vi "State Enter.vi"(8 "error in":errorcluster, 11 "State Pattern in":refnum<class "State Pattern.lvclass">) -> (0 "error out":errorcluster, 3 "State Pattern out":refnum<class "State Pattern.lvclass">)   [LabVIEW 2021, in "State Pattern.lvclass"]
uses:
  State Pattern.lvclass
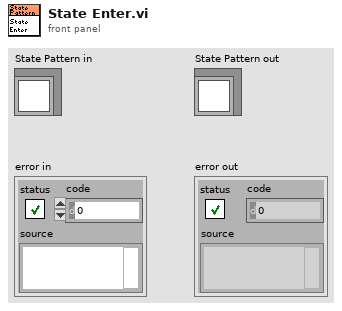
[diagram p1: front panel]
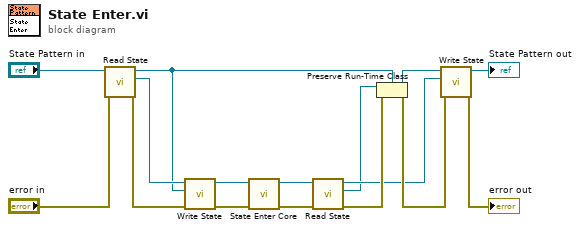
[diagram p0: block diagram]
diagram:
  n1 = call-dynamic "Read State.vi"("error in (no error)"="error in", "State Pattern in"="State Pattern in") -> ("error out"=w8:errorcluster, "State"=w14:refnum<class "State Pattern.lvclass">, "State Pattern out"=w10:refnum<class "State Pattern.lvclass">)  [unwired: 7 in]
  n2 = call-dynamic "Write State.vi"("error in (no error)"=w8, "State"=w10, "State Pattern in"=w14) -> ("error out"=w7:errorcluster, "State Pattern out"=w13:refnum<class "State Pattern.lvclass">)  [unwired: 7 in]
  n3 = call-dynamic "State Enter Core.vi"("error in (no error)"=w7, "State Pattern in"=w13) -> ("error out"=w6:errorcluster, "State Pattern out"=w12:refnum<class "State Pattern.lvclass">)  [unwired: 8 in]
  n4 = call-dynamic "Read State.vi"("error in (no error)"=w6, "State Pattern in"=w12) -> ("error out"=w5:errorcluster, "State"=w1:refnum<class "State Pattern.lvclass">, "State Pattern out"=w2:refnum<class "State Pattern.lvclass">)  [unwired: 7 in]
  n5 = Preserve Run-Time Class(object in=w1, error in=w5, 2:w10) -> (object out=w11:refnum<class "State Pattern.lvclass">, error out=w4:errorcluster)
  n6 = call-dynamic "Write State.vi"("error in (no error)"=w4, "State"=w2, "State Pattern in"=w11) -> ("error out"=→"error out":errorcluster, "State Pattern out"=→"State Pattern out":refnum<class "State Pattern.lvclass">)  [unwired: 7 in]
